vi "Login.vi"(0 "View Manager in":refnum<class "View Manager.lvclass">=refnum, 11 "error in (no error)":errorcluster) -> (4 "View Manager out":refnum<class "View Manager.lvclass">, 15 "error out":errorcluster)   [LabVIEW 2017, in "View Manager.lvlib" / "View Manager.lvclass"]
uses:
  View Manager.lvclass
  <vilib>/gpm_packages/@cs/mva-viewable/Source/IViewManager/IViewManager/IViewManager.lvclass
  <vilib>/gpm_packages/@cs/mva-viewable/Source/IViewable/IViewable Messages/Insert Front Panel Msg/Insert Front Panel Msg.lvclass
  C:/Program Files/National Instruments/LabVIEW 2017/vi.lib/gpm_packages/@cs/mva-viewable/Source/IViewable/IViewable/IViewable.lvclass
  C:/Program Files/National Instruments/LabVIEW 2017/vi.lib/gpm_packages/@cs/mva-viewable/Source/ActorEvents/IEventAggregator/IEventAggregator.lvclass
  C:/Program Files/National Instruments/LabVIEW 2017/vi.lib/gpm_packages/@cs/mva-core/Source/IObserver/IObserver/IObserver.lvclass
  C:/Program Files/National Instruments/LabVIEW 2017/vi.lib/ActorFramework/Actor/Actor.lvclass
  <vilib>/gpm_packages/@cs/mva-viewable/Source/IViewable/ProtectedSubpanel/ProtectedSubpanel.lvclass
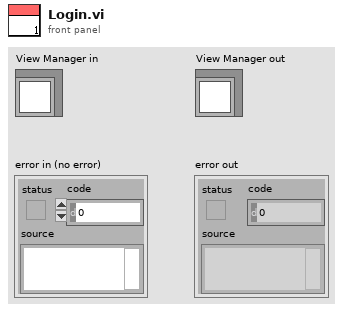
[diagram p1: front panel]
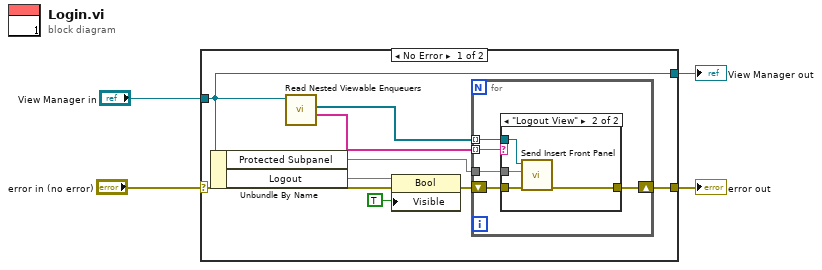
[diagram p0: block diagram]
diagram:
  n1 = case shown="No Error" "error in (no error)" {
    selector: "error in (no error)" -> [w7 w25]
    tunnel: [w6 w25] -> w3
    tunnel: [w10 w24] -> w1
    tunnel: "View Manager in" -> [w10 w24]
    frame No Error {
      n2 = Unbundle By Name(w10) -> ("Protected Subpanel"=w9, "Logout"=w5)
      n3 = call <vilib>:"Read Nested Viewable Enqueuers.vi"("IViewManager in"=w10) -> ("Viewable Names"=w11:string[], "Nested Viewable Enqueuers"=w12:refnum<class "Message Enqueuer.lvclass">[])  [unwired: 9 in]
      n4 = property class="Bool"(reference=w5, error in=w7, "Visible"=TRUE) -> (error out=w8:errorcluster)  [unwired: 1 out]
      n5 = for {
        tunnel: w12 -> [w18] mode=indexing
        tunnel: w11 -> [w17] mode=indexing
        tunnel: w9 -> [w16]
        shift-right: [w14] -> w6
        shift-left: w8 -> [w15]
        n6 = case shown="\"Logout View\"" w17 {
          tunnel: w18 -> [_ w23]
          tunnel: w16 -> [_ w22]
          tunnel: w15 -> [w19 w21]
          tunnel: [w19 w20] -> w14
          frame "False", Default {
          }
          frame "Logout View" {
            n7 = call <vilib>:"Send Insert Front Panel.vi"("error in (no error)"=w21, "Protected Subpanel"=w22, "Message Enqueuer"=w23) -> ("error out"=w20:errorcluster)  [unwired: 7 in, 1 out]
          }
        }
      }
    }
    frame Error {
    }
  }
  "error out" <- w3
  "View Manager out" <- w1
